vi "Append Waveform if new.vi"(8 "error in (no error)":errorcluster, 10 "New Waveform":waveform(dbl)[](array[waveform]), 11 "Waveforms in":waveform(dbl)[](array[waveform])) -> (0 "error out":errorcluster, 3 "AI Waveforms out":waveform(dbl)[](array[waveform]))   [LabVIEW 2019, in "SMO.Transport.lvclass"]
uses:
  SMO.Transport.lvclass
  <vilib>/Waveform/WDTOps.llb/WDT Append Waveforms DBL.vi
panel:
  out "t0 out":timestamp
  in  "t0 in":timestamp
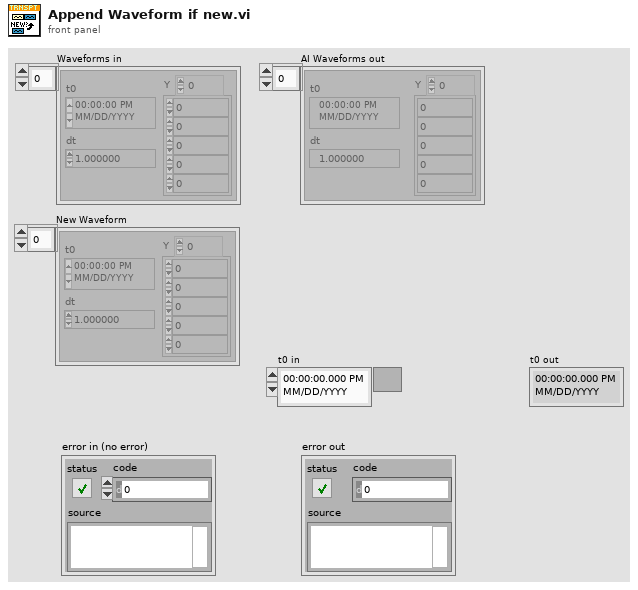
[diagram p1: front panel]
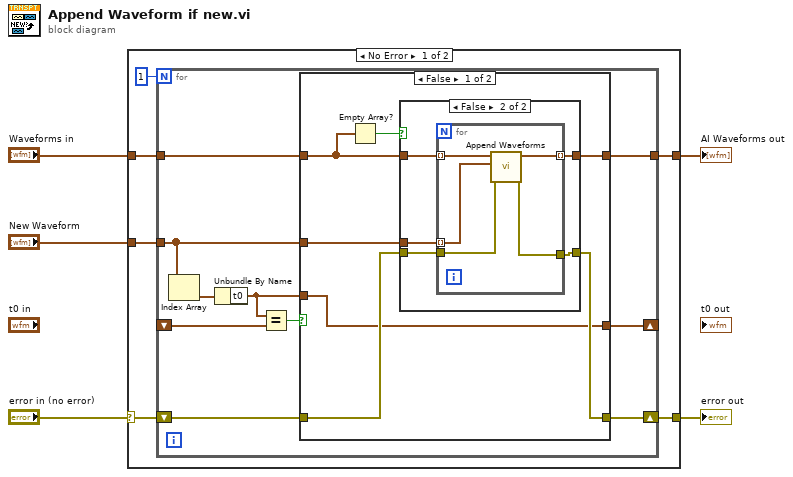
[diagram p0: block diagram]
diagram:
  n1 = case shown="No Error" "error in (no error)" {
    selector: "error in (no error)" -> [w8 w44]
    tunnel: "New Waveform" -> [w7 _]
    tunnel: [w11 w44] -> w4
    tunnel: [w10 w45] -> w3
    tunnel: "Waveforms in" -> [w9 w45]
    frame No Error {
      n2 = for {
        N: 1 -> [_]
        tunnel: [w17] -> w10
        tunnel: w9 -> [w16]
        tunnel: w7 -> [w12]
        shift-right: [w18] -> w11
        shift-left: w8 -> [w15]
        shift-right: [w21] -> _
        shift-left: _ -> [w13]
        n3 = Index Array(array=w12) -> (element=w19:waveform(dbl))  [unwired: 1 in]
        n4 = Unbundle By Name(w19) -> ("t0"=w14:timestamp)
        n5 = Equal?(x=w14, y=w13) -> (x = y?=w20:bool)
        n6 = case shown="False" w20 {
          tunnel: w16 -> [w23 w42]
          tunnel: [w27 w42] -> w17
          tunnel: [w26 w43] -> w18
          tunnel: w15 -> [w25 w43]
          tunnel: w12 -> [w28 _]
          tunnel: [w24 w41] -> w21
          tunnel: w14 -> [w24 w41]
          frame False {
            n7 = Empty Array?(array=w23) -> (empty?=w22:bool)
            n8 = case shown="False" w22 {
              tunnel: w28 -> [w30 w35]
              tunnel: [w30 w34] -> w27
              tunnel: [w29 w33] -> w26
              tunnel: w25 -> [w29 w31]
              tunnel: w23 -> [_ w32]
              frame True {
              }
              frame False {
                n9 = for {
                  tunnel: w32 -> [w38] mode=indexing
                  tunnel: w35 -> [w40] mode=indexing
                  tunnel: [w39] -> w34 mode=indexing
                  tunnel: [w36] -> w33
                  tunnel: w31 -> [w37]
                  n10 = call-poly <vilib>:"Append Waveforms.vi"("error in (no error)"=w37, "waveform B"=w40, "waveform A"=w38) -> ("error out"=w36:errorcluster, "waveform out"=w39:waveform(dbl))  [unwired: 7 in]
                }
              }
            }
          }
          frame True {
          }
        }
      }
    }
    frame Error {
    }
  }
  "error out" <- w4
  "AI Waveforms out" <- w3
